vi "Read (Single Point).vi"(0 "VISA resource name":refnum<visa-resource-name>, 1 "Timeout (100000ms)":u32=100000, 5 "Buffer Name (\"\")":string, 9 "Clear Buffer (No)":bool, 11 "error in (no error)":errorcluster) -> (4 "VISA resource name out":refnum<visa-resource-name>, 6 "Measurement":dbl, 15 "error out":errorcluster)   [LabVIEW 2020, in "Keithley DMM6500 DAQ6500 Series.lvlib"]
doc: "Gets a simple read from instrument."
uses:
  <instrlib>/Keithley DMM6500 DAQ6500 Series/Keithley DMM6500 DAQ6500 Series.lvlib
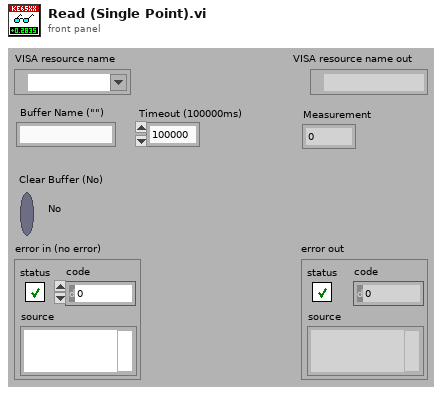
[diagram p1: front panel]
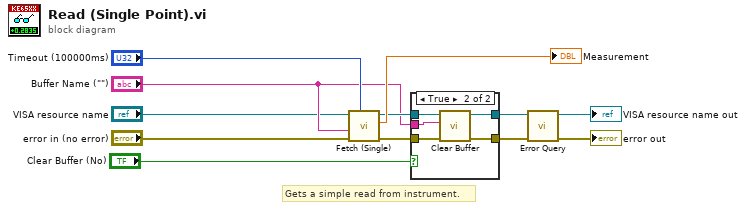
[diagram p0: block diagram]
diagram:
  # "Gets a simple read from instrument."
  n1 = call <instrlib>:"Fetch (Single).vi"("Timeout (100000ms)"="Timeout (100000ms)", "error in (no error)"="error in (no error)", "Buffer Name ()"="Buffer Name (\"\")", "VISA resource name"="VISA resource name") -> ("error out"=w9:errorcluster, "Output Value"=→"Measurement":dbl, "VISA resource name out"=w10:refnum<visa-resource-name>)  [unwired: 5 in]
  n2 = case shown="True" "Clear Buffer (No)" {
    tunnel: w10 -> [w14 w19]
    tunnel: [w14 w18] -> w5
    tunnel: w9 -> [w13 w17]
    tunnel: [w13 w16] -> w3
    tunnel: "Buffer Name (\"\")" -> [_ w15]
    frame False {
    }
    frame True {
      n3 = call <instrlib>:"Clear Buffer.vi"("error in (no error)"=w17, "Buffer Name (\"\")"=w15, "VISA resource name"=w19) -> ("error out"=w16:errorcluster, "VISA resource name out"=w18:refnum<visa-resource-name>)  [unwired: 7 in]
    }
  }
  n4 = call <instrlib>:"Error Query.vi"("error in (no error)"=w3, "VISA resource name"=w5) -> ("error out"=→"error out":errorcluster, "VISA resource name out"=→"VISA resource name out":refnum<visa-resource-name>)  [unwired: 6 in, 2 out]
